vi "Disconnect from Slave.vi"(8 "error in":errorcluster, 11 "TCP master in":refnum<class "TCP.lvclass">) -> (0 "error out":errorcluster, 3 "TCP master out":refnum<class "TCP.lvclass">)   [LabVIEW 2021, in "TCP.lvclass"]
doc: "Closes the TCP connection stored in the class."
uses:
  TCP.lvclass
  TCP.lvclass/TCP.ctl
  Transmission Data Unit/Transmission Data Unit.lvclass
  Network Master/Network Master.lvclass
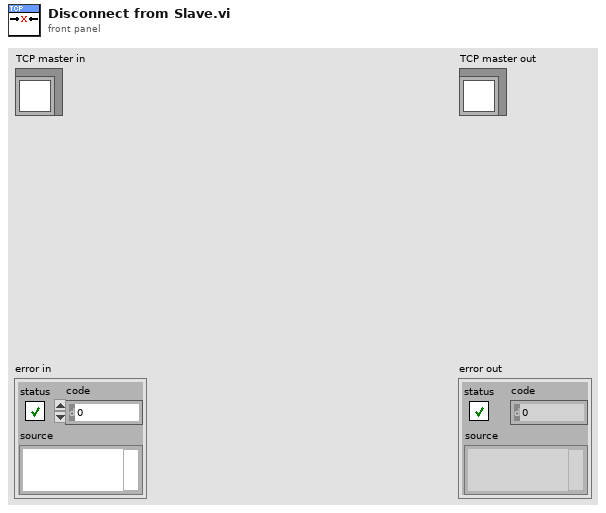
[diagram p1: front panel]
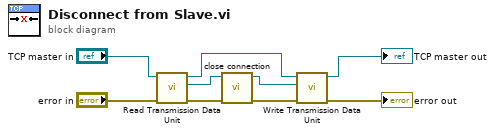
[diagram p0: block diagram]
diagram:
  n1 = call "Read Transmission Data Unit.vi"("error in (no error)"="error in", "Network Master in"="TCP master in") -> ("error out"=w4:errorcluster, "Transmission Data Unit"=w2:refnum<class "Transmission Data Unit.lvclass">, "Network Master out"=w5:refnum<class "TCP.lvclass">)  [unwired: 7 in]
  n2 = call-dynamic "close connection.vi"("error in"=w4, "transmission data unit in"=w2) -> ("error out"=w3:errorcluster, "transmission data unit out"=w1:refnum<class "Transmission Data Unit.lvclass">)  [unwired: 8 in]
  n3 = call "Write Transmission Data Unit.vi"("error in (no error)"=w3, "Transmission Data Unit"=w1, "Network Master in"=w5) -> ("error out"=→"error out":errorcluster, "Network Master out"=→"TCP master out":refnum<class "TCP.lvclass">)  [unwired: 7 in]
